vi "Unregister Event(All Events In Customize Register).vi"(8 "error in (no error)":errorcluster, 11 "Register Name":string) -> (0 "error out":errorcluster)   [LabVIEW 2019, in "FootScan Engine Event.lvlib"]
uses:
  FootScan Engine Event.lvlib
  <userlib>/JUL/Event Message Module/Event Message Library/Event Action.ctl
panel:
  # "Input"
  # "Output"
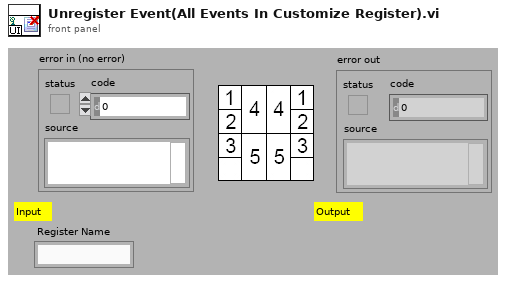
[diagram p1: front panel]
types:
  T1 = typedef "Event Action.ctl" = enum16{"Default", "Generate Event", "Register", "Unregister(Customize Event and Register)", "Unregister(All Events In Customize Register)", "Unregister(All Registers In Customize Event)", "Get Register Table"}
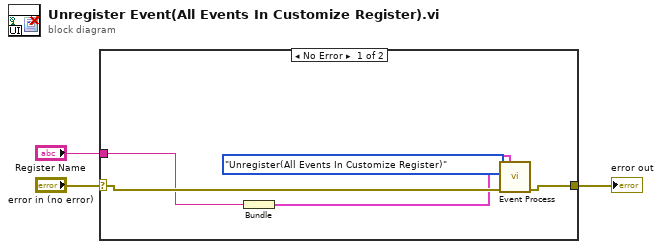
[diagram p0: block diagram]
diagram:
  n1 = case shown="No Error" "error in (no error)" {
    selector: "error in (no error)" -> [w7 w9]
    tunnel: [w6 w9] -> w1
    tunnel: "Register Name" -> [w5 _]
    frame No Error {
      n2 = Bundle("Register Name"=w5) -> (w4:cluster{"Register Name":string})  [unwired: 1 in]
      n3 = call "Event Process.vi"("Event Action"=Event_Action."Unregister(All Events In Customize Register)", "Unregister Event Data(All Events In Customize Register)"=w4, "error in (no error)"=w7) -> ("error out"=w6:errorcluster)  [unwired: 11 in, 1 out]
    }
    frame Error {
    }
  }
  "error out" <- w1
